vi "Read Section Names.vi"(8 "error in (no error)":errorcluster, 11 "Ini-File in":refnum<class "Ini-File.lvclass">) -> (0 "error out":errorcluster, 1 "Section Names":string[](array[string]), 2 "Section Classes":path[](array[path]), 3 "Ini-File out":refnum<class "Ini-File.lvclass">)   [LabVIEW 2015, in "Configuration.lvlib" / "Ini-File.lvclass"]
doc: "Read available sections and pathes to corresponding derived class of Sections.lvclass."
uses:
  Ini-File.lvclass
  Ini-File.lvclass/Ini-File.ctl
  <vilib>/Utility/config.llb/Read Key (Path).vi
  <vilib>/Utility/config.llb/NI_LVConfig.lvlib
  Configuration/Configuration.lvclass
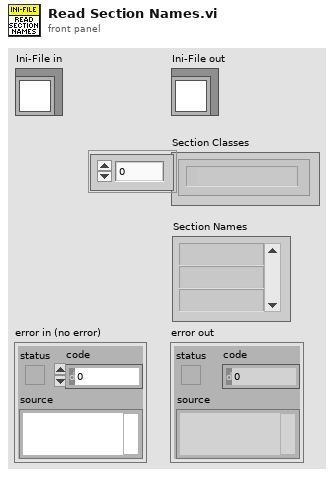
[diagram p1: front panel]
types:
  T1 = typedef "NI_LVConfig.lvlib/Config Data RefNum.ctl" = refnum<k1>
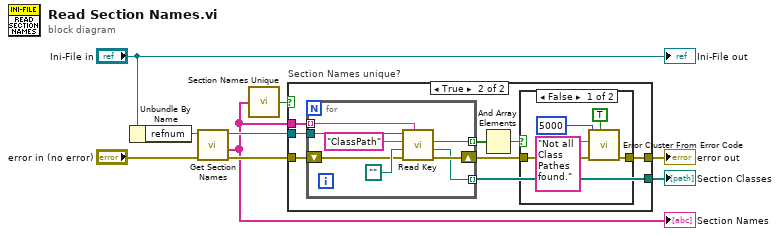
[diagram p0: block diagram]
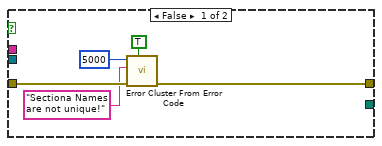
[diagram p2: hidden frame]
diagram:
  n1 = Unbundle By Name("Ini-File in") -> ("refnum"=w3:T1)
  n2 = call <vilib>:"Get Section Names.vi"("error in (no error)"="error in (no error)", "refnum"=w3) -> ("error out"=w8:errorcluster, "section names"=w6:string[], "refnum out"=w7:T1)  [unwired: 7 in]
  "Section Names" <- w6
  n3 = call "Section Names Unique.vi"("Section Names"=w6) -> ("Unique?"=w5:bool)
  n4 = case "Section Names unique?" shown="True" w5 {
    tunnel: [_ w22] -> w9
    tunnel: w8 -> [w12 w21]
    tunnel: w7 -> [_ w20]
    tunnel: [w11 w16] -> w1
    tunnel: w6 -> [_ w19]
    frame False {
      n5 = call <vilib>:"Error Cluster From Error Code.vi"("show call chain? (False)"=TRUE, "error in (no error)"=w12, "error message (\"\")"="Sectiona Names are not unique!" ("error message (\"\")"), "error code (0)"=5000) -> ("error out"=w11:errorcluster)  [unwired: 5 in]
    }
    frame True {
      n6 = for {
        tunnel: w19 -> [w35] mode=indexing
        tunnel: [w30] -> w22 mode=indexing
        shift-right: [w31] -> w17
        shift-left: w21 -> [w32]
        tunnel: w20 -> [w36]
        tunnel: [w29] -> w18 mode=indexing
        n7 = call-poly <vilib>:"Read Key.vi"("section"=w35, "error in (no error)"=w32, "default value"=path "", "key"="ClassPath", "refnum"=w36) -> ("error out"=w31:errorcluster, "value"=w30:path, "found?"=w29:bool)  [unwired: 3 in, 1 out]
      }
      n8 = And Array Elements(Boolean array=w18) -> (logical AND=w15:bool)
      n9 = case shown="False" w15 {
        tunnel: w17 -> [w27 w28]
        tunnel: [w26 w28] -> w16
        frame False {
          n10 = call <vilib>:"Error Cluster From Error Code.vi"("show call chain? (False)"=TRUE, "error in (no error)"=w27, "error message (\"\")"="Not all Class Pathes found." ("error message (\"\")"), "error code (0)"=5000) -> ("error out"=w26:errorcluster)  [unwired: 5 in]
        }
        frame True {
        }
      }
    }
  }
  "error out" <- w1
  "Section Classes" <- w9
  "Ini-File out" <- "Ini-File in"
